vi "auto-range_on-off.vi"() -> ()   [LabVIEW 2024]
panel:
  in  "Auto-Range":bool
  in  "error-in":errorcluster
  in  "VISA-in":refnum<visa-resource-name>
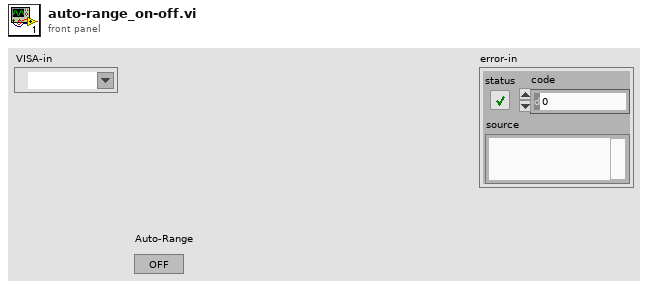
[diagram p1: front panel]
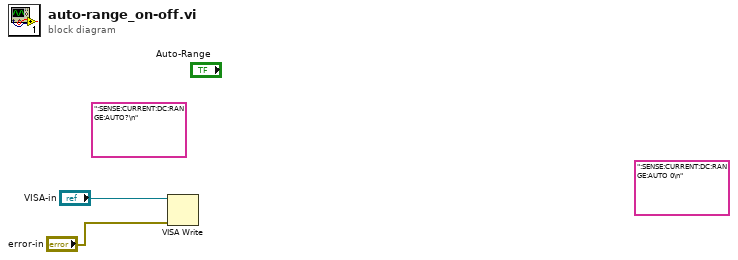
[diagram p0: block diagram]
diagram:
  (unwired) ":SENSE:CURRENT:DC:RANGE:AUTO 0\n"
  (unwired) ":SENSE:CURRENT:DC:RANGE:AUTO?\n"
  n1 = VISA Write(VISA resource name="VISA-in", error in (no error)="error-in") -> ()  [unwired: 1 in, 3 out]
